vi "获取标点符号(冲突时的文件备份2013-05-03 10-12-13).vi"() -> ()   [LabVIEW 2012]
panel:
  out "标点符号":u16(ring)=8
  out "标点符号":u16(ring)=8
  out "标点符号":string[](array[string])=["　", "，", "、", "。", "．", "；", "：", "？", "！", "︰", "…", "‥", "′", "‵", "々", "～", "‖", "ˇ", "ˉ", "﹐", "﹑", "﹒", "·", "﹔", "﹕", "﹖", "﹗", "｜", "︱", "︳", "︴", "﹏", "（", "）", "︵", "︵", "｛", "｝", "︷", "︸", "〔", "〕", "︹", "︺", "【", "】", "︻", "︼", "《", "》", "︽", "︾", "〈", "〉", "︿", "﹀", "「", "」", "﹁", "﹂", "﹁", "『", "』", "﹂", "﹃", "﹄", "﹙", "﹚", "〝", "〞", "ˋ", "ˊ"]
  in  "WORD粘贴标点符号字符串":string="　 ， 、 。 ． ； ： ？ ！ ︰ … ‥ ′ ‵ 々 ～ ‖ ˇ ˉ ﹐ ﹑ ﹒ · ﹔ ﹕ ﹖ ﹗ ｜ ︱ ︳ ︴ ﹏ （ ） ︵ ︵ ｛ ｝ ︷ ︸ 〔 〕 ︹ ︺ 【 】 ︻ ︼ 《 》 ︽ ︾ 〈 〉 ︿ ﹀ 「 」 ﹁ ﹂ ﹁ 『 』 ﹂ ﹃ ﹄ ﹙ ﹚ 〝 〞 ˋ ˊ"
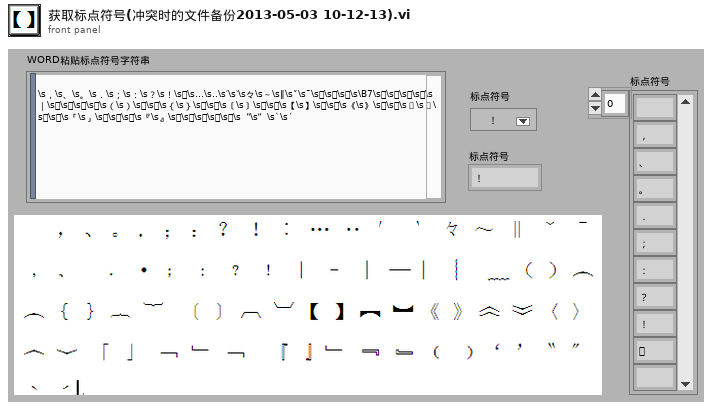
[diagram p1: front panel]
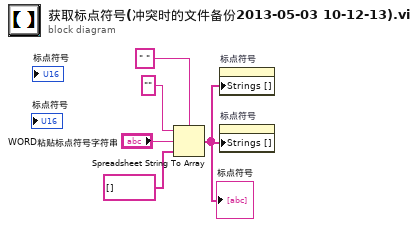
[diagram p0: block diagram]
diagram:
  n1 = Spreadsheet String To Array(delimiter (Tab)=" " ("分隔符(Tab)"), format string="" ("格式字符串"), spreadsheet string="WORD粘贴标点符号字符串", array type (2D Dbl)=string[] []) -> (array=w1:string[])
  "标点符号" <- w1
  n2 = property on="标点符号" class="Ring (严格)"("Strings []"=w1) -> ()  [unwired: 2 in, 2 out]
  n3 = property on="标点符号" class="Ring (严格)"("Strings []"=w1) -> ()  [unwired: 2 in, 2 out]
